vi "windowed and unwindowed signal.vi"() -> ()   [LabVIEW 2009]
uses:
  <vilib>/Analysis/4window.llb/Hamming Window (DBL).vi
  <vilib>/Analysis/NI_AALBase.lvlib
  <vilib>/Analysis/NI_AALPro.lvlib
panel:
  out "?":string="When the number of cycles is set to an integral number, the spectrum of the windowed signal is broader (wider) than the spectrum of the nonwindowed signal."
  in  "stop":bool
  in  "CYCLES":dbl=19.0
  out "SPECTRUM OF WINDOWED SIGNAL":dbl[](graph)=[2.9099816902921457e-18, 8.85499560561452e-18, 1.583043785580593e-18, 1.241645053050708e-17, 8.544551844076658e-18, 5.374168851108688e-18, 4.5745100841095464e-18, 1.7141327880896493e-19, 6.212988452357125e-18, 1.3091728647434963e-17, 5.453501646609877e-18, 9.479820326812426e-18, 1.3738024455592368e-18, 2.5272912410716758e-17, 1.3222813275165959e-17, 1.3920714458451346e-17, 9.97766908989755e-18, 1.618984355384205e-17, 0.16263455967290621, 0.3818376618407357, 0.16263455967290577, 2.422054618922019e-17, 7.624213224283211e-18, 7.700352261886636e-18, 8.698024986268852e-18, 7.617565564555194e-18, 1.8789971544685134e-17, 3.6623472579922254e-18, 1.163569064029759e-17, 7.218407950081517e-18, 9.123373976904062e-18, 3.574975142996534e-18, 7.175871589357373e-18, 7.059869829621427e-18, 2.668095177298236e-18, 8.340522098957292e-18, 2.4336030302381524e-18, 7.110438598077492e-18, 5.5732171157377916e-18, 4.46795099621482e-18, 4.458905780839609e-18, 5.1024438741843886e-18, 9.779941621004778e-18, 5.841781630938393e-18, 8.909484784391497e-18, 4.1675936515959226e-17, 6.561430834106298e-18, 2.4940062431513334e-18, 2.663879618360171e-18, 5.3727900195627905e-18, 3.694253352726616e-18, 2.5272912410716758e-17, 1.251734928089371e-17, 8.324459090651482e-18, 4.0837668804811196e-19, 4.7416392728812795e-18, 1.6626336560032565e-18, 5.201682162357824e-18, 3.428509089495198e-18, 1.1111679406372346e-17, 9.816528809806176e-19, 1.527793305110782e-17, 1.1253522420937535e-18, 3.1936564795671635e-18]
  out "WINDOWED SIGNAL":dbl[](graph)=[0.0, 0.06470165189653335, 0.07867487432505382, 0.02862849729810987, -0.0493561767137086, -0.09367265463964201, -0.06331717317481252, 0.025972085829052898, 0.10626038788318887, 0.10649980867103312, 0.013165291627424906, -0.10776751743040852, -0.1544971992672426, -0.07290863371594025, 0.0869327194721522, 0.19700684919375788, 0.15183766184073577, -0.03390690073394827, -0.2188744162068062, -0.24044155342282836, -0.05549104108401945, 0.20382669689317315, 0.3216014093645072, 0.17650414832424324, -0.13928361315005414, -0.37349178085474627, -0.3142048234302635, 0.021012206862470347, 0.37437622041443896, 0.4448833197925615, 0.14366540370226316, -0.3082320178697577, -0.54, -0.33512323098207053, 0.16984204773255607, 0.571984270605101, 0.5236109608723103, 0.031980881411141575, -0.5206464662014922, -0.6741419725953616, -0.27401449380424353, 0.37872681540443565, 0.7531980954414654, 0.5214569743416075, -0.15520650669339806, -0.7358668831504902, -0.733600549289418, -0.12456201167784375, 0.6118376618407346, 0.871303781568206, 0.4221757562999267, -0.38885086718876305, -0.9047509035682462, -0.6924596979529487, 0.09269321992849876, 0.8198470901292599, 0.8915295072290017, 0.23644650846647408, -0.6218275737219231, -0.9850264380619445, -0.5506596749474637, 0.33521254436548575, 0.9548206882657312, 0.8027624821025646, 2.326752072262517e-15, -0.8027624821025618, -0.9548206882657326, -0.33521254436549014, 0.5506596749474598, 0.9850264380619442, 0.6218275737219268, -0.23644650846646967, -0.891529507229, -0.8198470901292623, -0.09269321992850314, 0.6924596979529456, 0.904750903568247, 0.3888508671887669, -0.42217575629992304, -0.8713037815682054, -0.6118376618407375, 0.12456201167783984, 0.7336005492894161, 0.7358668831504918, 0.15520650669340172, -0.5214569743416049, -0.7531980954414658, -0.3787268154044386, 0.2740144938042405, 0.6741419725953608, 0.5206464662014941, -0.03198088141113854, -0.5236109608723086, -0.5719842706051019, -0.16984204773255868, 0.3351232309820684, 0.54, 0.3082320178697596, -0.14366540370226097, -0.4448833197925608, -0.3743762204144401, -0.021012206862472335, 0.3142048234302623, 0.3734917808547467, 0.13928361315005572, -0.17650414832424186, -0.3216014093645071, -0.2038266968931742, 0.05549104108401816, 0.24044155342282783, 0.21887441620680675, 0.03390690073394933, -0.15183766184073508, -0.197006849193758, -0.08693271947215296, 0.07290863371593953, 0.15449719926724245, 0.10776751743040898, -0.013165291627424284, -0.10649980867103283, -0.10626038788318908, -0.025972085829053377, 0.06331717317481214, 0.09367265463964204, 0.04935617671370895, -0.028628497298109495, -0.07867487432505371, -0.06470165189653357]
  out "SPECTRUM OF ORIGINAL SIGNAL":dbl[](graph)=[1.7798279804180986e-17, 2.8061208126825453e-17, 2.674182123623628e-17, 3.693287134529762e-17, 2.996148197212313e-17, 1.862495926619565e-17, 3.606555036857666e-17, 3.426366092080452e-17, 3.6180558457816035e-17, 4.743494512143997e-17, 5.1450128176592155e-17, 5.791654235294668e-17, 6.445149110994305e-17, 5.06713729866171e-17, 9.361408931420286e-17, 1.1994224942426323e-16, 1.6518580416126984e-16, 2.5463109622033016e-16, 5.1196102012833e-16, 0.7071067811865476, 5.337582427329305e-16, 2.6053105625638413e-16, 1.8294609566727506e-16, 1.3104745109023214e-16, 1.110845082765646e-16, 1.0514946071008348e-16, 8.432945637545613e-17, 8.399249542152345e-17, 6.670530337301702e-17, 5.633809487892007e-17, 5.399369877993352e-17, 4.682575814481787e-17, 5.181973316402492e-17, 5.596285978711425e-17, 4.5733416152141676e-17, 2.5836544404667057e-17, 4.211038304111686e-17, 3.935072533548419e-17, 3.946340061568668e-17, 2.6981494973893346e-17, 3.355753602951269e-17, 3.628849453766811e-17, 3.33390663048306e-17, 3.899189242531141e-17, 3.168866977953073e-17, 7.978638829519201e-17, 2.8867974652844825e-17, 3.223942930023381e-17, 2.78420168050082e-17, 3.398219186096461e-17, 2.947772096886307e-17, 1.1461544172371152e-16, 2.794918271455769e-17, 2.9214018781333316e-17, 2.5321488982839292e-17, 2.939685127477217e-17, 2.315131438234518e-17, 3.1077600230153767e-17, 2.4288275750688415e-17, 3.3648006015510317e-17, 2.6778065754489192e-17, 3.250637249051996e-17, 2.3055583362012716e-17, 3.066883254565195e-17]
  out "ORIGINAL SIGNAL":dbl[](graph)=[0.0, 0.8032075314806449, 0.9569403357322089, 0.33688985339222016, -0.5555702330196021, -0.9987954562051724, -0.6343932841636457, 0.24298017990326365, 0.9238795325112866, 0.8577286100002722, 0.09801714032956096, -0.7409511253549588, -0.9807852804032305, -0.42755509343028253, 0.4713967368259972, 0.9891765099647809, 0.7071067811865479, -0.14673047445536114, -0.8819212643483547, -0.9039892931234437, -0.19509032201612897, 0.6715589548470179, 0.9951847266721969, 0.5141027441932224, -0.38268343236508895, -0.9700312531945438, -0.7730104533627375, 0.04906767432741704, 0.8314696123025447, 0.9415440651830211, 0.2902846772544634, -0.5956993044924325, -1.0, -0.5956993044924344, 0.29028467725446117, 0.9415440651830204, 0.831469612302546, 0.04906767432741936, -0.7730104533627361, -0.9700312531945443, -0.3826834323650911, 0.5141027441932204, 0.9951847266721967, 0.6715589548470196, -0.1950903220161267, -0.9039892931234427, -0.8819212643483558, -0.14673047445536344, 0.7071067811865462, 0.9891765099647812, 0.47139673682599925, -0.4275550934302804, -0.9807852804032301, -0.7409511253549604, 0.09801714032955865, 0.857728610000271, 0.9238795325112875, 0.2429801799032659, -0.6343932841636438, -0.9987954562051725, -0.5555702330196041, 0.33688985339221794, 0.9569403357322082, 0.8032075314806463, 2.3267520722625168e-15, -0.8032075314806435, -0.9569403357322096, -0.3368898533922223, 0.5555702330196002, 0.9987954562051723, 0.6343932841636475, -0.24298017990326137, -0.9238795325112857, -0.8577286100002735, -0.09801714032956328, 0.7409511253549572, 0.980785280403231, 0.42755509343028464, -0.47139673682599514, -0.9891765099647806, -0.7071067811865496, 0.14673047445535883, 0.8819212643483536, 0.9039892931234447, 0.19509032201613127, -0.6715589548470161, -0.9951847266721972, -0.5141027441932244, 0.38268343236508684, 0.9700312531945432, 0.773010453362739, -0.04906767432741471, -0.8314696123025433, -0.9415440651830219, -0.29028467725446566, 0.5956993044924306, 1.0, 0.5956993044924361, -0.29028467725445894, -0.9415440651830196, -0.8314696123025472, -0.04906767432742168, 0.7730104533627347, 0.9700312531945449, 0.3826834323650933, -0.5141027441932184, -0.9951847266721965, -0.6715589548470213, 0.19509032201612442, 0.9039892931234417, 0.8819212643483569, 0.14673047445536574, -0.7071067811865447, -0.9891765099647816, -0.4713967368260013, 0.4275550934302783, 0.9807852804032297, 0.740951125354962, -0.09801714032955633, -0.8577286100002699, -0.9238795325112884, -0.24298017990326815, 0.634393284163642, 0.9987954562051726, 0.555570233019606, -0.3368898533922158, -0.9569403357322075, -0.8032075314806476]
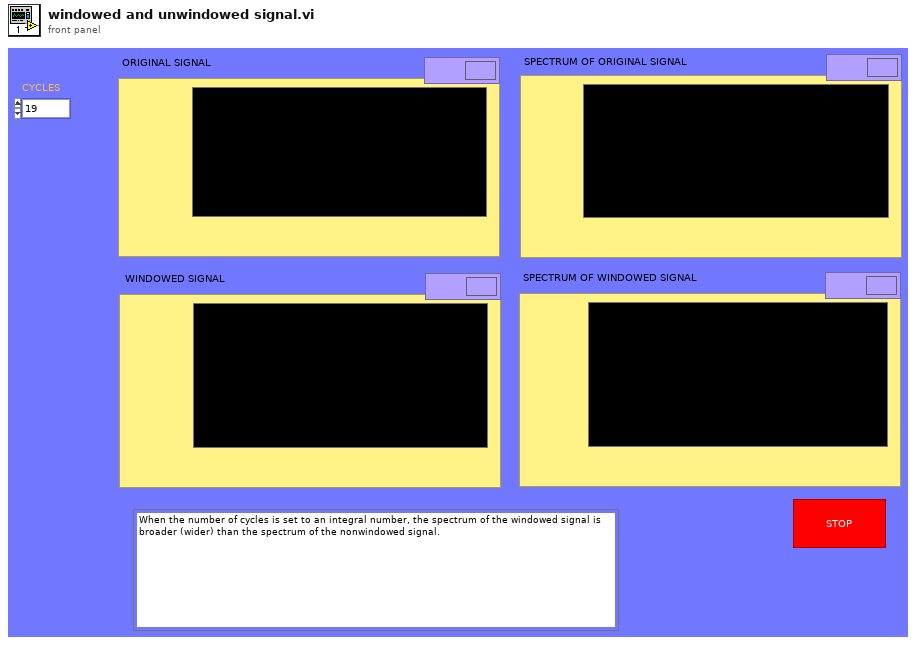
[diagram p1: front panel]
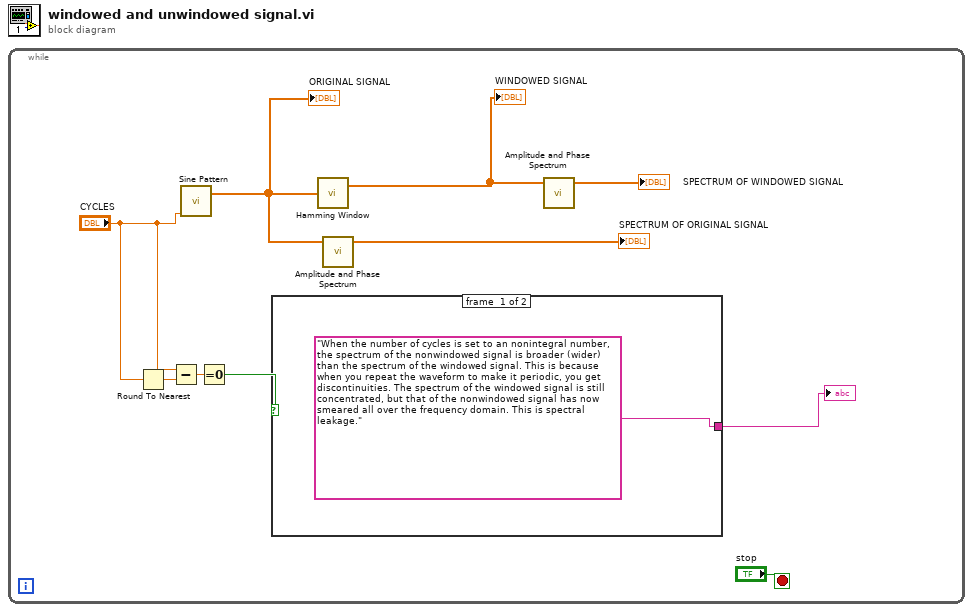
[diagram p0: block diagram]
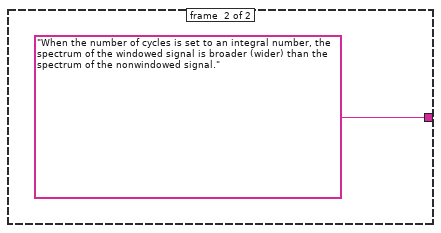
[diagram p2: hidden frame]
diagram:
  n1 = while {
    stop <- "stop" stop-if-true
    n2 = Round To Nearest(number="CYCLES") -> (nearest integer value=w5:dbl)
    n3 = Subtract(x="CYCLES", y=w5) -> (x-y=w3:dbl)
    n4 = call <vilib>:"Sine Pattern.vi"("cycles"="CYCLES") -> ("Sinusoidal Pattern"=w10:dbl[])  [unwired: 3 in, 1 out]
    "ORIGINAL SIGNAL" <- w10
    n5 = Equal To 0?(x=w3) -> (x = 0?=w2:bool)
    n6 = case shown="False" w2 {
      tunnel: ["When the number of cycles is set to an nonintegral number, the spectrum of the nonwindowed signal is broader (wider) than the spectrum of the windowed signal. This is because when you repeat the waveform to make it periodic, you get discontinuities. The spectrum of the windowed signal is still concentrated, but that of the nonwindowed signal has now smeared all over the frequency domain. This is spectral leakage." "When the number of cycles is set to an integral number, the spectrum of the windowed signal is broader (wider) than the spectrum of the nonwindowed signal."] -> w1
      frame #0 {
      }
      frame #1 {
      }
    }
    "?" <- w1
    n7 = call-poly <vilib>:"Hamming Window.vi"("X"=w10) -> ("Windowed X"=w8:dbl[])  [unwired: 1 out]
    "WINDOWED SIGNAL" <- w8
    n8 = call <vilib>:"Amplitude and Phase Spectrum.vi"("Signal (V)"=w10) -> ("Amp Spectrum Mag (Vrms)"=→"SPECTRUM OF ORIGINAL SIGNAL":dbl[])  [unwired: 2 in, 2 out]
    n9 = call <vilib>:"Amplitude and Phase Spectrum.vi"("Signal (V)"=w8) -> ("Amp Spectrum Mag (Vrms)"=→"SPECTRUM OF WINDOWED SIGNAL":dbl[])  [unwired: 2 in, 2 out]
  }
